vi "Main.vi"(10 "WHL Panel":refnum<vi>, 11 "Module Admin":refnum<class "Delacor_lib_QMH_Module Admin.lvclass">) -> ()   [LabVIEW 2019, in "TIME STAMP.lvlib"]
doc: "This template is based off of the Queued Message Handler design pattern and the Queued Message Handler project template that ships with LabVIEW.\n\nThe main difference is that the queue is private to this module and communication between modules is performed via Broadcast and Request events.\n\nRequest events are wrapped in public API methods and are handled in the Event Handling Loop (EHL) of this VI. Any module can register for Broadcast events sent by this module. The EHL generates messages based on user interface actions.\n\nThe Message Handling Loop (MHL) processes messages generated by the EHL, or by other messages. The messages are string values, so new messages can be added easily to the Message Cases case structure in the MHL. Each message cluster can also provide an optional value for Message Data, which is a variant that can be converted to whatever message-specific data is required.\n_____\nBased on Delacor QMH Project Template 5.0.0.82."
uses:
  TIME STAMP.lvlib
  <vilib>/Delacor/Delacor QMH/Libraries/Module Admin_class/Delacor_lib_QMH_Module Admin.lvclass
  Module Data--cluster.ctl
  STOP HELPER LOOP Argument--cluster.ctl
  Stop Argument--cluster.ctl
  <vilib>/Delacor/Delacor QMH/Libraries/Message Queue_class/Delacor_lib_QMH_Message Queue.lvclass/Delacor_lib_QMH_Message Queue.ctl
  <vilib>/Delacor/Delacor QMH/Libraries/Module Admin_class/Delacor_lib_QMH_Module Admin.lvclass/Delacor_lib_QMH_Module Admin.ctl
  <vilib>/Utility/miscctls.llb/LVPointTypeDef.ctl
  <vilib>/Delacor/Delacor QMH/Libraries/Message Queue_class/Delacor_lib_QMH_Enqueue Message (Single).vi
  <vilib>/Delacor/Delacor QMH/Libraries/Module Admin_class/Delacor_lib_QMH_Get External Launch.vi
  <vilib>/Utility/error.llb/Error Cluster From Error Code.vi
  <vilib>/ErrorRing/Error Ring.xnode
  <vilib>/Delacor/Delacor QMH/Libraries/Message Queue_class/Delacor_lib_QMH_Message Queue.lvclass
panel:
  out "Time stamp":timestamp
  out "error out":errorcluster
  out "Status":string
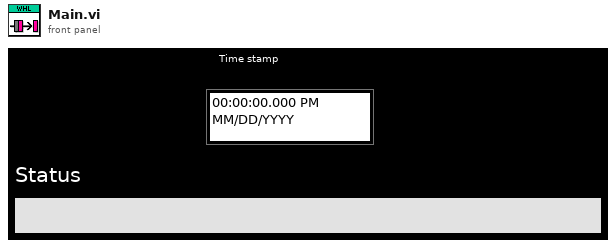
[diagram p1: front panel]
types:
  T1 = typedef "TIME STAMP.lvlib/Request Events--cluster.ctl" = cluster{"Stop Module":refnum<user-event>, "Show Panel":refnum<user-event>, "Hide Panel":refnum<user-event>, "Get Module Execution Status":refnum<user-event>, "Show Diagram":refnum<user-event>, "START HELPER LOOP":refnum<user-event>, "STOP HELPER LOOP":refnum<user-event>}
  T2 = typedef "TIME STAMP.lvlib/Module Data--cluster.ctl" = cluster{"Status":string}
  T3 = typedef "TIME STAMP.lvlib/STOP HELPER LOOP Argument--cluster.ctl" = cluster{"Boolean":bool}
  T4 = enum32{"invalid lock state", "Not Locked", "Locked (No Password)", "Password-protected"}
  T5 = typedef "TIME STAMP.lvlib/Stop Argument--cluster.ctl" = cluster{"Origin":string, "Exit via Stop Module Req?":bool, "Wait for Module to stop?":bool}
  T6 = typedef "LVPointTypeDef.ctl" = cluster{"Horizontal":i16, "Vertical":i16}
  T7 = enum32{"Invalid", "Standard", "Closed", "Hidden", "Minimized", "Maximized"}
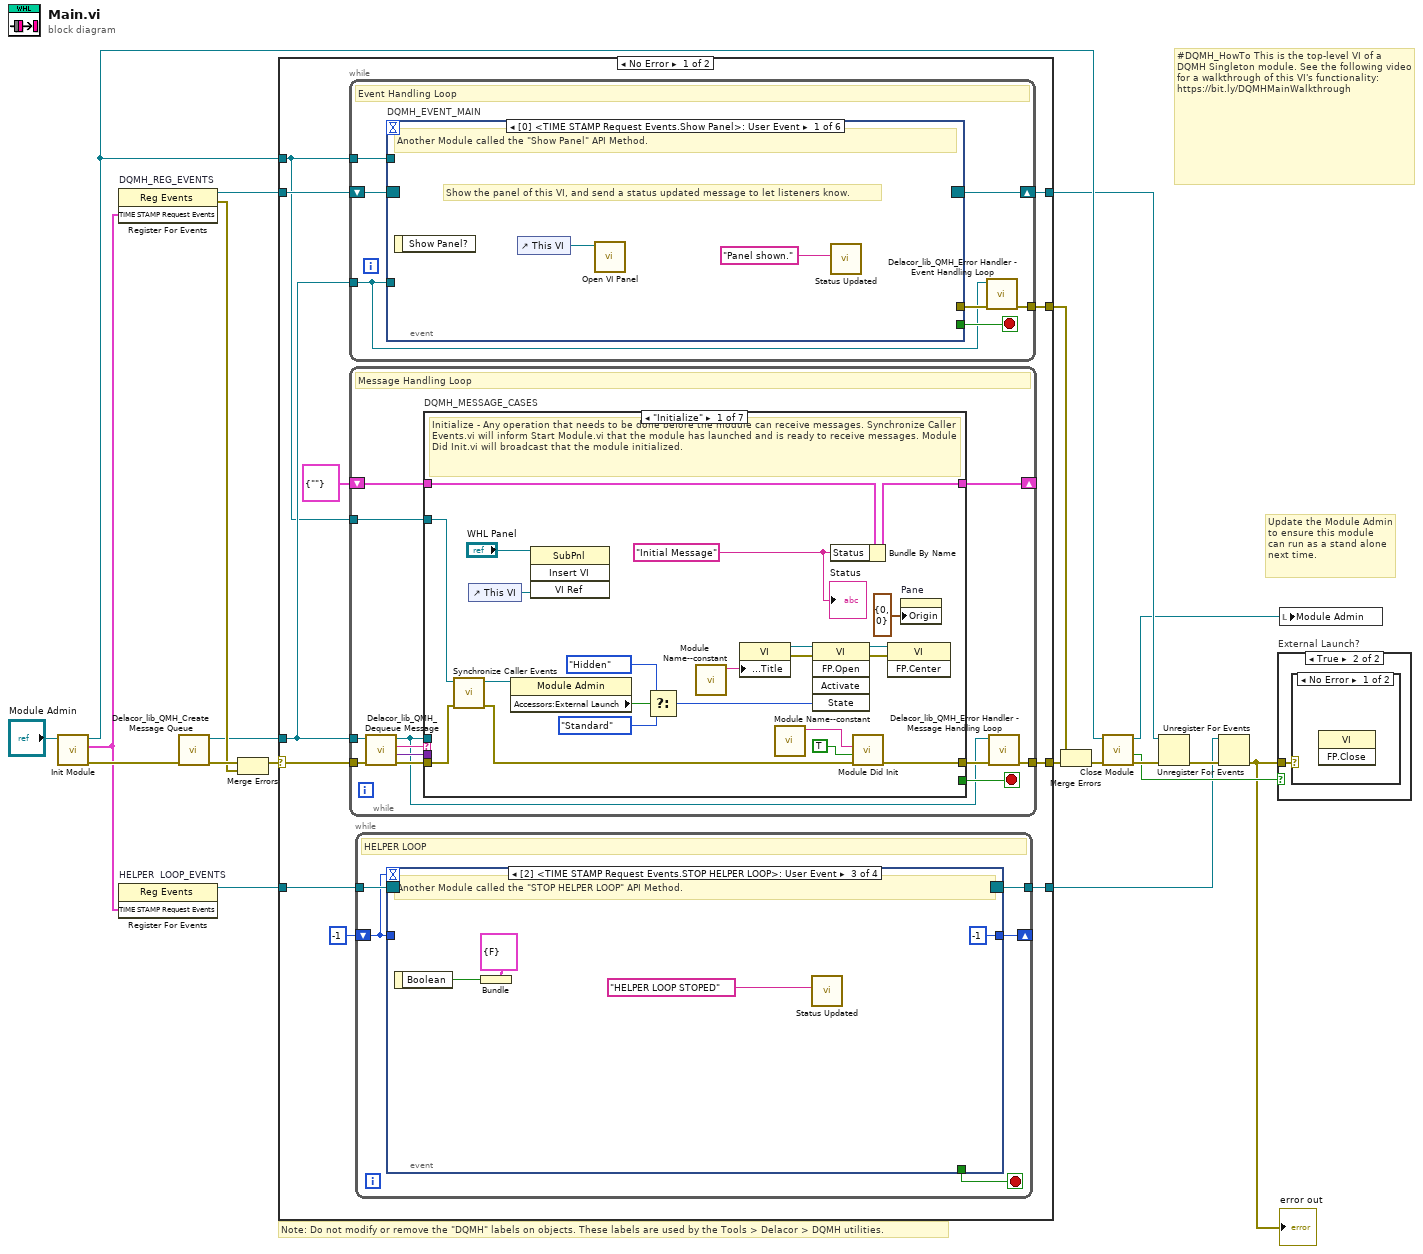
[diagram p0: block diagram]
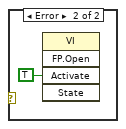
[diagram p3: hidden frame]
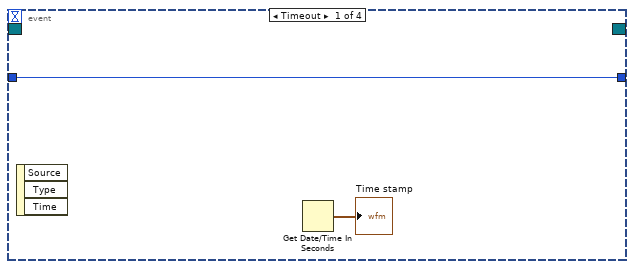
[diagram p4: hidden frame]
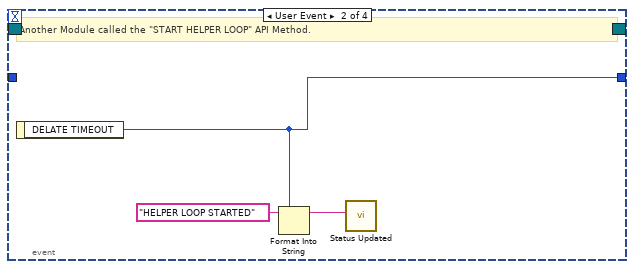
[diagram p5: hidden frame]
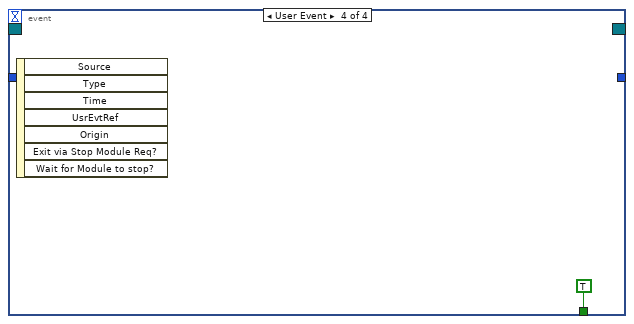
[diagram p6: hidden frame]
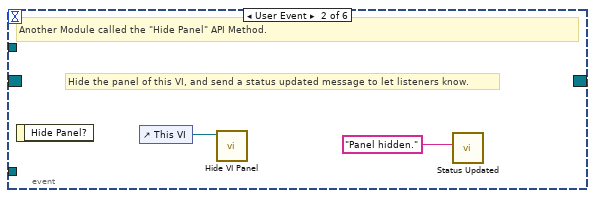
[diagram p7: hidden frame]
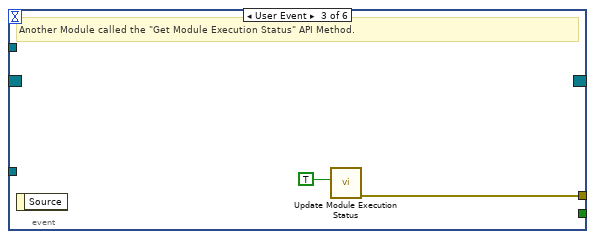
[diagram p8: hidden frame]
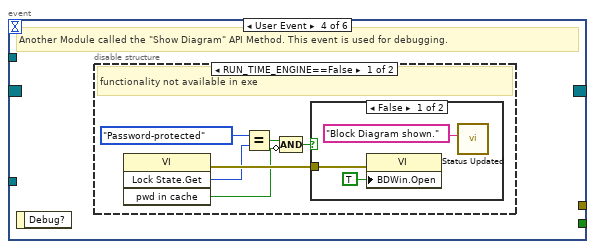
[diagram p9: hidden frame]
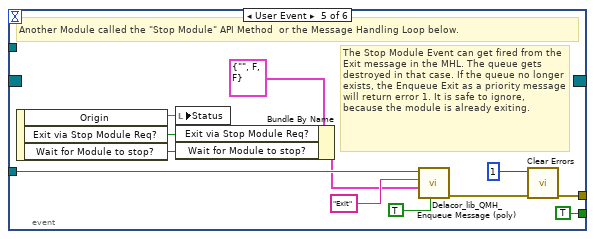
[diagram p12: hidden frame]
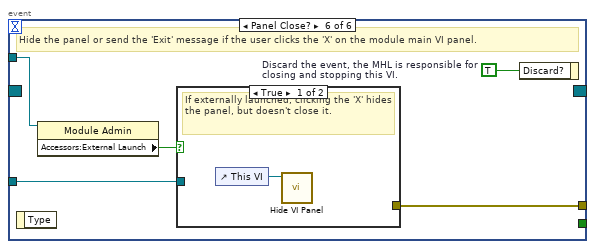
[diagram p13: hidden frame]
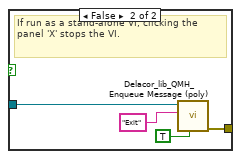
[diagram p14: hidden frame]
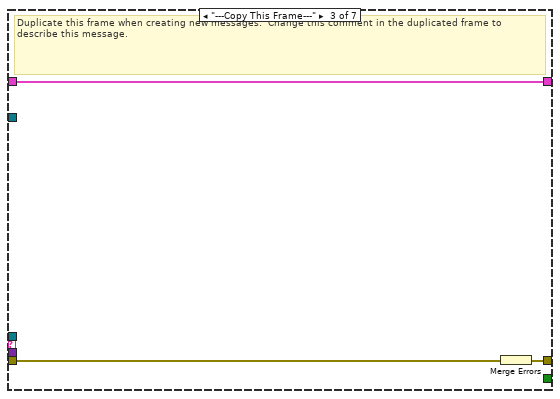
[diagram p16: hidden frame]
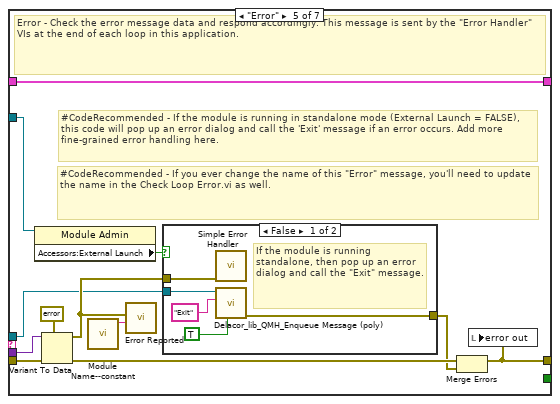
[diagram p18: hidden frame]
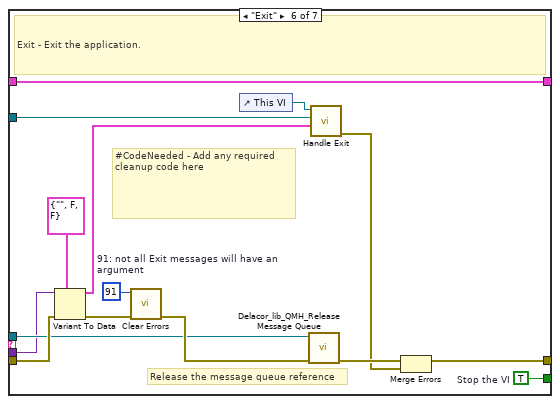
[diagram p20: hidden frame]
diagram:
  # "#DQMH_HowTo This is the top-level VI of a DQMH Singleton module. See the following video for a walkthrough of this VI's functionality: https://bit.ly/DQMHMainWalkthrough"
  # "Note: Do not modify or remove the \"DQMH\" labels on objects. These labels are used by the Tools > Delacor > DQMH utilities."
  # "Update the Module Admin to ensure this module can run as a stand alone next time."
  n1 = call "Init Module.vi"("Singleton Module Admin in"="Module Admin") -> ("error out"=w19:errorcluster, "TIME STAMP Request Events"=w5:T1, "Singleton Module Admin out"=w12:refnum<class "Delacor_lib_QMH_Module Admin.lvclass">)  [unwired: 8 in]
  n2 = register-events "DQMH_REG_EVENTS"(w5) -> (reference out=w10:refnum<event-registration>, error out=w13:errorcluster)  [unwired: 2 in]
  n3 = register-events "HELPER  LOOP_EVENTS"(w5) -> (reference out=w4:refnum<event-registration>)  [unwired: 2 in, 1 out]
  n4 = call <vilib>:"Delacor_lib_QMH_Create Message Queue.vi"("error in (no error)"=w19) -> ("error out"=w15:errorcluster, "Message Queue"=w9:refnum<class "Delacor_lib_QMH_Message Queue.lvclass">)  [unwired: 9 in]
  n5 = Merge Errors(w15, w13) -> (w14:errorcluster)
  n6 = case shown="No Error" w14 {
    selector: w14 -> [w29 w181]
    tunnel: [w31 w180] -> w20
    tunnel: [w28 w186] -> w11
    tunnel: w10 -> [w26 w186]
    tunnel: w9 -> [w25 w179]
    tunnel: [w30 _] -> w17
    tunnel: w12 -> [w24 w182]
    tunnel: w4 -> [w23 w178]
    tunnel: [w22 w178] -> w1
    frame No Error {
      n7 = while {
        tunnel: w25 -> [w47]
        shift-right: [w50] -> w28
        shift-left: w26 -> [w51]
        tunnel: [w52] -> w30
        tunnel: w24 -> [w48]
        stop <- w49 stop-if-true
        # "Event Handling Loop"
        n8 = event "DQMH_EVENT_MAIN" shown="[0] <TIME STAMP Request Events.Show Panel>: User Event" {
          selector: w51 -> [_ _ _ _ _ _]
          dyn-events: [_ _ _ _ _ _] -> w50
          timeout: _ -> [_ _ _ _ _ _]
          tunnel: [_ _ _ _ TRUE ("Discard?") _] -> w49
          tunnel: w47 -> [_ _ _ _ w76 w83]
          tunnel: [_ _ w59 _ w79 w85] -> w53
          tunnel: w48 -> [_ _ _ _ _ w82]
          event User Event {
            # "Show the panel of this VI, and send a status updated message to let listeners know."
            # "Another Module called the \"Show Panel\" API Method."
            n9 = event-data() -> ()  [unwired: 1 in, 1 out]
            n10 = control-ref of="This VI"() -> (w55:refnum<vi>)
            n11 = call "Open VI Panel.vi"("VI"=w55) -> ()  [unwired: 10 in, 1 out]
            n12 = call "Status Updated.vi"("Status"="Panel shown." ("format string")) -> ()  [unwired: 10 in, 1 out]
          }
          event User Event {
            # "Hide the panel of this VI, and send a status updated message to let listeners know."
            # "Another Module called the \"Hide Panel\" API Method."
            n13 = event-data() -> ()  [unwired: 1 in, 1 out]
            n14 = control-ref of="This VI"() -> (w57:refnum<vi>)
            n15 = call "Hide VI Panel.vi"("VI"=w57) -> ()  [unwired: 10 in, 1 out]
            n16 = call "Status Updated.vi"("Status"="Panel hidden." ("format string")) -> ()  [unwired: 10 in, 1 out]
          }
          event User Event {
            # "Another Module called the \"Get Module Execution Status\" API Method."
            n17 = event-data() -> ()  [unwired: 1 in, 1 out]
            n18 = call "Update Module Execution Status.vi"("Running?"=TRUE) -> ("error out"=w59:errorcluster)  [unwired: 10 in]
          }
          event User Event {
            # "Another Module called the \"Show Diagram\" API Method. This event is used for debugging."
            n19 = event-data() -> ()  [unwired: 1 in, 1 out]
            n20 = disable-structure shown="RUN_TIME_ENGINE==False" {
              frame condition #0 (active) {
                # "functionality not available in exe"
                n21 = invoke class="VI" method="Lock State.Get"() -> (error out=w65:errorcluster, "Get Lock State"=w64:T4, "pwd in cache"=w61:bool)  [unwired: 4 in, 1 out]
                n22 = Equal?(x=T4."Password-protected", y=w64) -> (x = y?=w62:bool)
                n23 = Compound Arithmetic op=AND(w62, invert w61) -> (w60:bool)
                n24 = case shown="False" w60 {
                  tunnel: w65 -> [w68 _]
                  frame False {
                    n25 = property class="VI"(error in=w68, "BDWin.Open"=TRUE ("Block Diagram Window:Open")) -> ()  [unwired: 1 in, 2 out]
                    n26 = call "Status Updated.vi"("Status"="Block Diagram shown." ("format string")) -> ()  [unwired: 10 in, 1 out]
                  }
                  frame True {
                    # "Password-protected VI, and the password is not in the cache. Do not show the diagram."
                  }
                }
              }
              frame condition #1 {
              }
            }
          }
          event User Event {
            # "The Stop Module Event can get fired from the Exit message in the MHL. The queue gets destroyed in that case. If the queue no longer exists, the Enqueue Exit as a priority message will return error 1. It is safe to ignore, because the module is already exiting."
            # "Another Module called the \"Stop Module\" API Method  or the Message Handling Loop below."
            n27 = event-data() -> ("Origin"=w75:string, "Exit via Stop Module Req?"=w71:bool, "Wait for Module to stop?"=w70:bool)  [unwired: 1 in]
            n28 = local write "Status"(w75) -> ()
            n29 = Bundle By Name(cluster=T5 {"Origin"="", "Exit via Stop Module Req?"=FALSE, "Wait for Module to stop?"=FALSE} ("Stop Argument"), "Exit via Stop Module Req?"=w71, "Wait for Module to stop?"=w70) -> (w69:T5)
            n30 = call-poly <vilib>:"Delacor_lib_QMH_Enqueue Message (poly).vi"("Priority Message? (F)"=TRUE, "Message Data"=w69, "Message"="Exit", "Message Queue in"=w76) -> ("error out"=w80:errorcluster)  [unwired: 6 in, 1 out]
            n31 = call <vilib>:"Clear Errors.vi"("error in (no error)"=w80, "specific error code to clear (0: all)"=1) -> ("error out"=w79:errorcluster)  [unwired: 4 in, 1 out]
          }
          event Panel Close? {
            w84 = TRUE  # Discard the event, the MHL is responsible for closing and stopping this VI.
            # "Hide the panel or send the 'Exit' message if the user clicks the 'X' on the module main VI panel."
            n32 = event-data() -> ()  [unwired: 1 in, 1 out]
            n33 = property class="Module Admin"(reference=w82) -> ("Accessors:External Launch"=w81:bool)  [unwired: 1 in, 2 out]
            n34 = case shown="True" w81 {
              tunnel: w83 -> [_ w89]
              tunnel: [_ w90] -> w85
              frame True {
                # "If externally launched, clicking the 'X' hides the panel, but doesn't close it."
                n35 = control-ref of="This VI"() -> (w86:refnum<vi>)
                n36 = call "Hide VI Panel.vi"("VI"=w86) -> ()  [unwired: 10 in, 1 out]
              }
              frame False {
                # "If run as a stand-alone VI, clicking the panel 'X' stops the VI."
                n37 = call-poly <vilib>:"Delacor_lib_QMH_Enqueue Message (poly).vi"("Priority Message? (F)"=TRUE, "Message"="Exit", "Message Queue in"=w89) -> ("error out"=w90:errorcluster)  [unwired: 7 in, 1 out]
              }
            }
            n38 = event-data("Discard?"=w84) -> ()  [unwired: 1 in, 1 out]
          }
        }
        n39 = call-dynamic "Delacor_lib_QMH_Error Handler - Event Handling Loop.vi"("error in (no error)"=w53, "Message Queue in"=w47) -> ("dup error in"=w52:errorcluster)  [unwired: 8 in, 1 out]
      }
      n40 = while {
        tunnel: w25 -> [w93]
        shift-right: [w97] -> _
        shift-left: T2 {"Status"=""} ("Data Cluster") -> [w98]
        tunnel: w29 -> [w101]
        tunnel: [w99] -> w31
        tunnel: w24 -> [w91]
        stop <- w96 stop-if-true
        # "Message Handling Loop"
        n41 = call-dynamic "Delacor_lib_QMH_Dequeue Message.vi"("error in (no error)"=w101, "Message Queue in"=w93) -> ("error out"=w100:errorcluster, "Message Data"=w94:variant, "Message"=w95:string, "Message Queue out"=w92:refnum<class "Delacor_lib_QMH_Message Queue.lvclass">)  [unwired: 6 in]
        n42 = case "DQMH_MESSAGE_CASES" shown="\"Initialize\"" w95 {
          selector: w95 -> [_ _ _ _ _ _ w165]
          tunnel: w92 -> [_ _ _ _ w135 w157 _]
          tunnel: w100 -> [w122 w126 w129 w131 w142 w163 w167]
          tunnel: [w120 w126 w128 w131 w138 w160 w168] -> w102
          tunnel: w98 -> [w111 w125 w127 w130 w137 w156 w166]
          tunnel: [w110 w125 w127 w130 w137 w156 w166] -> w97
          tunnel: [_ _ _ _ _ w155 _] -> w96
          tunnel: w94 -> [_ _ _ _ w136 w154 _]
          tunnel: w91 -> [w112 _ _ _ w134 w149 _]
          frame "Initialize" {
            w105 = "Initial Message" ("Initial Message")
            # "Initialize - Any operation that needs to be done before the module can receive messages. Synchronize Caller Events.vi will inform Start Module.vi that the module has launched and is ready to receive messages. Module Did Init.vi will broadcast that the module initialized."
            n43 = call "Synchronize Caller Events.vi"("error in (no error)"=w122, "Singleton Module Admin in"=w112) -> ("error out"=w121:errorcluster, "Singleton Module Admin out"=w107:refnum<class "Delacor_lib_QMH_Module Admin.lvclass">)  [unwired: 8 in]
            n44 = control-ref of="This VI"() -> (w103:refnum<vi>)
            n45 = property class="Module Admin"(reference=w107) -> ("Accessors:External Launch"=w116:bool)  [unwired: 1 in, 2 out]
            n46 = invoke class="SubPnl" method="Insert VI"(reference="WHL Panel", "VI Ref"=w103) -> ()  [unwired: 2 in, 4 out]
            n47 = Select(t=T7."Hidden" ("State"), s=w116, f=T7."Standard" ("State")) -> (s? t:f=w113:T7)
            n48 = call "Module Name--constant.vi"() -> ("Module Name"=w119:string)  [unwired: 11 in]
            n49 = property class="VI"("Front Panel.Title"=w119) -> (reference out=w118:refnum<vi>, error out=w124:errorcluster)  [unwired: 2 in]
            n50 = call "Module Name--constant.vi"() -> ("Module Name"=w108:string)  [unwired: 11 in]
            n51 = invoke class="VI" method="FP.Open"(reference=w118, error in=w124, "State"=w113) -> (reference out=w117:refnum<vi>, error out=w123:errorcluster)  [unwired: 2 in, 3 out]
            n52 = Bundle By Name(cluster=w111, "Status"=w105) -> (w110:T2)
            n53 = call "Module Did Init.vi"("error in (no error)"=w121, "Initialized?"=TRUE, "Origin"=w108) -> ("error out"=w120:errorcluster)  [unwired: 8 in]
            n54 = invoke class="VI" method="FP.Center"(reference=w117, error in=w123) -> ()  [unwired: 1 in, 3 out]
            n55 = property on="Pane" class="Pane"("Origin"=T6 {"Horizontal"=0, "Vertical"=0}) -> ()  [unwired: 2 in, 2 out]
            "Status" <- w105
          }
          frame "--- Module Specific ---" {
            # "Separator -- The following cases handle messages specific to this Module."
          }
          frame "---Copy This Frame---" {
            # "Duplicate this frame when creating new messages.  Change this comment in the duplicated frame to describe this message."
            n56 = Merge Errors(w129) -> (w128:errorcluster)
          }
          frame "--- Exit and Error Handling---" {
            # "Separator - The following cases handle errors and exit messages."
          }
          frame "Error" {
            # "#CodeRecommended - If you ever change the name of this \"Error\" message, you'll need to update the name in the Check Loop Error.vi as well."
            # "#CodeRecommended - If the module is running in standalone mode (External Launch = FALSE), this code will pop up an error dialog and call the 'Exit' message if an error occurs. Add more fine-grained error handling here."
            # "Error - Check the error message data and respond accordingly. This message is sent by the \"Error Handler\" VIs at the end of each loop in this application."
            n57 = property class="Module Admin"(reference=w134) -> ("Accessors:External Launch"=w133:bool)  [unwired: 1 in, 2 out]
            n58 = Variant To Data(error in=w142, type=errorcluster {"status"=FALSE, "code"=0, "source"=""} ("error constant"), Variant=w136) -> (data=w143:errorcluster, error out=w140:errorcluster)
            n59 = call "Module Name--constant.vi"() -> ("Module Name"=w132:string)  [unwired: 11 in]
            n60 = call "Error Reported.vi"("Additional Information"=w132, "Error"=w143) -> ()  [unwired: 9 in, 1 out]
            n61 = case shown="False" w133 {
              tunnel: [w148 _] -> w139
              tunnel: w135 -> [w146 _]
              tunnel: w143 -> [w147 _]
              frame False {
                # "If the module is running standalone, then pop up an error dialog and call the \"Exit\" message."
                n62 = call <vilib>:"Simple Error Handler.vi"("error in (no error)"=w147) -> ()  [unwired: 4 in, 5 out]
                n63 = call-poly <vilib>:"Delacor_lib_QMH_Enqueue Message (poly).vi"("Priority Message? (F)"=TRUE, "Message"="Exit", "Message Queue in"=w146) -> ("error out"=w148:errorcluster)  [unwired: 7 in, 1 out]
              }
              frame True {
                # "If the module was launched externally, calling the Error Reported broadcast VI is the only action performed by the \"Error\" message. The module's caller can then process the error appropriately."
              }
            }
            n64 = Merge Errors(w140, w139) -> (w138:errorcluster)
            n65 = local write "error out"(w138) -> ()
          }
          frame "Exit" {
            w153 = 91  # 91: not all Exit messages will have an argument
            w155 = TRUE  # Stop the VI
            # "Release the message queue reference"
            # "#CodeNeeded - Add any required cleanup code here"
            # "Exit - Exit the application."
            n66 = Variant To Data(error in=w163, type=T5 {"Origin"="", "Exit via Stop Module Req?"=FALSE, "Wait for Module to stop?"=FALSE} ("Stop Argument"), Variant=w154) -> (data=w151:T5, error out=w159:errorcluster)
            n67 = call <vilib>:"Clear Errors.vi"("error in (no error)"=w159, "specific error code to clear (0: all)"=w153) -> ("error out"=w162:errorcluster)  [unwired: 4 in, 1 out]
            n68 = control-ref of="This VI"() -> (w150:refnum<vi>)
            n69 = call-dynamic "Delacor_lib_QMH_Release Message Queue.vi"("error in (no error)"=w162, "Message Queue"=w157) -> ("error out"=w161:errorcluster)  [unwired: 9 in]
            n70 = call "Handle Exit.vi"("Stop Argument"=w151, "Admin in"=w149, "VI reference"=w150) -> ("error out"=w158:errorcluster)  [unwired: 7 in, 1 out]
            n71 = Merge Errors(w161, w158) -> (w160:errorcluster)
          }
          frame Default {
            # "'Default' case only runs if there is a message that isn't defined in any of the other cases.  Output a programming error."
            n72 = call "Module Name--constant.vi"() -> ("Module Name"=w164:string)  [unwired: 11 in]
            n73 = xnode "Error Ring"("parameter 0"=w165, "parameter 1"=w164) -> ("error out"=w169:errorcluster)
            n74 = Merge Errors(w167, w169) -> (w168:errorcluster)
          }
        }
        n75 = call-dynamic "Delacor_lib_QMH_Error Handler - Message Handling Loop.vi"("error in (no error)"=w102, "Message Queue in"=w92) -> ("dup error in"=w99:errorcluster)  [unwired: 8 in, 1 out]
      }
      n76 = while {
        tunnel: w23 -> [w36]
        tunnel: [w35] -> w22
        shift-right: [w33] -> _
        shift-left: -1 -> [w32]
        stop <- w34 stop-if-true
        # "HELPER LOOP"
        n77 = event shown="[2] <TIME STAMP Request Events.STOP HELPER LOOP>: User Event" {
          selector: w36 -> [_ _ _ _]
          dyn-events: [_ _ _ _] -> w35
          timeout: w32 -> [_ _ _ _]
          tunnel: [_ _ _ TRUE] -> w34
          tunnel: [w38 w40 -1 _] -> w33
          tunnel: w32 -> [w38 _ _ _]
          event Timeout {
            n78 = event-data() -> ()  [unwired: 1 in, 3 out]
            n79 = Get Date/Time In Seconds() -> (seconds since 1Jan1904=→"Time stamp":timestamp)
          }
          event User Event {
            # "Another Module called the \"START HELPER LOOP\" API Method."
            n80 = event-data() -> ("DELATE TIMEOUT"=w40:i32)  [unwired: 1 in]
            n81 = Format Into String(initial string="HELPER LOOP STARTED", w40) -> (resulting string=w41:string)  [unwired: 2 in, 1 out]
            n82 = call "Status Updated.vi"("Status"=w41) -> ()  [unwired: 10 in, 1 out]
          }
          event User Event {
            # "Another Module called the \"STOP HELPER LOOP\" API Method."
            n83 = event-data() -> ("Boolean"=w45:bool)  [unwired: 1 in]
            n84 = Bundle(cluster=T3 {"Boolean"=FALSE} ("STOP HELPER LOOP Argument"), "Boolean"=w45) -> ()  [unwired: 1 out]
            n85 = call "Status Updated.vi"("Status"="HELPER LOOP STOPED" ("initial string")) -> ()  [unwired: 10 in, 1 out]
          }
          event User Event {
            n86 = event-data() -> ()  [unwired: 1 in, 7 out]
          }
        }
      }
    }
    frame Error {
      # "Synchronize Caller Events.vi will inform Start Module.vi that the module has launched and will let the code calling Start Module.vi register for broadcasts and would permit the caller receive the broadcast that an error occurred at launch time."
      n87 = call-dynamic "Delacor_lib_QMH_Release Message Queue.vi"("error in (no error)"=w181, "Message Queue"=w179) -> ("error out"=w180:errorcluster)  [unwired: 9 in]
      n88 = call "Synchronize Caller Events.vi"("Singleton Module Admin in"=w182) -> ("error out"=w187:errorcluster)  [unwired: 9 in, 1 out]
      n89 = call "Module Name--constant.vi"() -> ("Module Name"=w185:string)  [unwired: 11 in]
      n90 = Format Into String(format string="An error occurred during initialization. %s is no longer running.", w185) -> (resulting string=w183:string)  [unwired: 2 in, 1 out]
      n91 = Merge Errors(w180, w187) -> (w188:errorcluster)
      n92 = call "Error Reported.vi"("Additional Information"=w183, "Error"=w188) -> ()  [unwired: 9 in, 1 out]
    }
  }
  n93 = Merge Errors(w17, w20) -> (w16:errorcluster)
  n94 = call "Close Module.vi"("error in (no error)"=w16, "Module Admin in"=w12) -> ("error out"=w18:errorcluster, "External Launch"=w6:bool, "Module Admin out"=w7:refnum<class "Delacor_lib_QMH_Module Admin.lvclass">)  [unwired: 7 in]
  n95 = Unregister For Events(event registration refnum=w11, error in=w18) -> (error out=w3:errorcluster)
  n96 = Unregister For Events(event registration refnum=w1, error in=w3) -> (error out=w2:errorcluster)
  "error out" <- w2
  n97 = case "External Launch?" shown="True" w6 {
    tunnel: w2 -> [_ w189]
    frame False {
    }
    frame True {
      n98 = case shown="No Error" w189 {
        frame No Error {
          n99 = invoke class="VI" method="FP.Close"() -> ()  [unwired: 3 in, 3 out]
        }
        frame Error {
          n100 = invoke class="VI" method="FP.Open"("Activate"=TRUE ("Activate?")) -> ()  [unwired: 4 in, 5 out]
        }
      }
    }
  }
  n101 = local write "Module Admin"(w7) -> ()
